vi "String to 1D Array 2.vi"(8 "Enum":T1(ring), 10 "string":string) -> (2 "Array of Strings":string[](array[string])=["sin(x)+2", "VIA(x", "y)", " VIB(z)"])   [LabVIEW 2017]
uses:
  <userlib>/_NEVSTOP/Communicable State Machine(CSM)/Communicable State Machine.lvlib
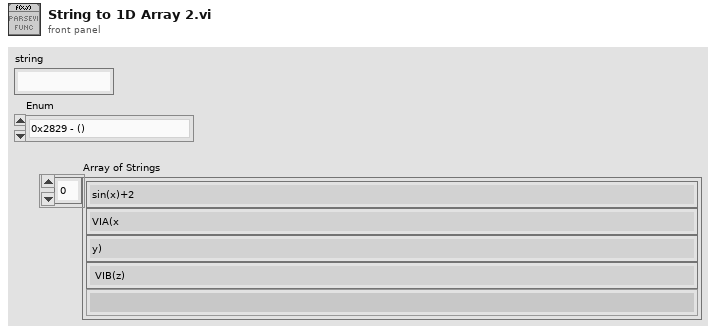
[diagram p1: front panel]
types:
  T1 = enum16{"0x2829 - ()", "0x5B5D - []", "0x7B7D - {}"}
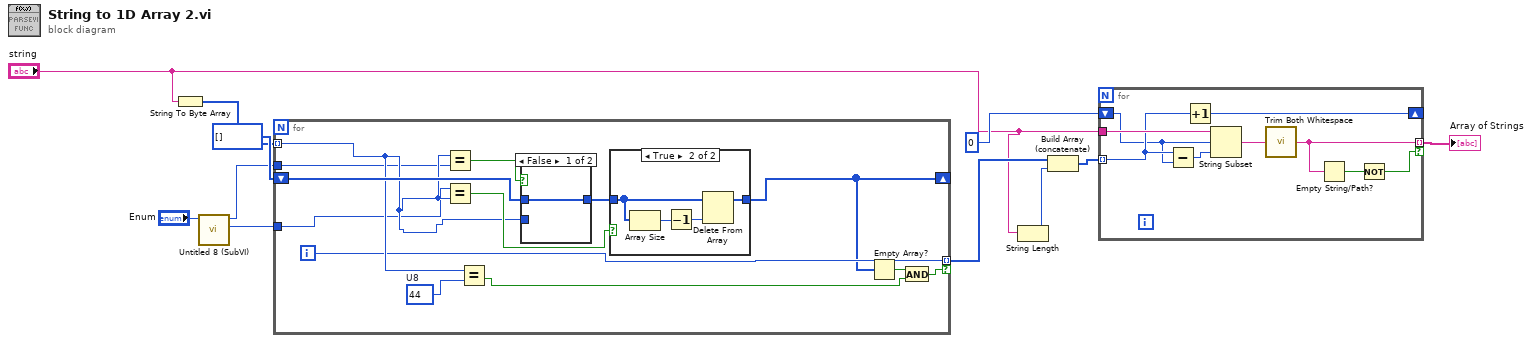
[diagram p0: block diagram]
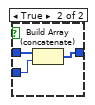
[diagram p3: hidden frame]
diagram:
  n1 = String To Byte Array(string="string") -> (unsigned byte array=w10:u8[])
  n2 = call "Untitled 8 (SubVI).vi"("Enum"="Enum") -> ("Numeric"=w1:u8, "Numeric 2"=w2:u8)  [unwired: 9 in]
  n3 = for {
    tunnel: w10 -> [w19] mode=indexing
    shift-right: [w16] -> _
    shift-left: i32[] [] -> [w21]
    tunnel: [w18] -> w9 mode=indexing if=w15
    tunnel: w2 -> [w13]
    tunnel: w1 -> [w12]
    i -> [w18]
    w20 = u8 44  # U8
    n4 = Equal?(x=w19, y=w13) -> (x = y?=w24:bool)
    n5 = Equal?(x=w12, y=w19) -> (x = y?=w22:bool)
    n6 = Equal?(x=w19, y=w20) -> (x = y?=w14:bool)
    n7 = case shown="False" w24 {
      tunnel: w21 -> [w30 w33]
      tunnel: w19 -> [_ w32]
      tunnel: [w30 w31] -> w23
      frame False {
      }
      frame True {
        n8 = Build Array (concatenate)(w33, w32) -> (w31:i32[])
      }
    }
    n9 = case shown="True" w22 {
      tunnel: w23 -> [w25 w28]
      tunnel: [w25 w26] -> w16
      frame False {
      }
      frame True {
        n10 = Array Size(array=w28) -> (size(s)=w29:i32)
        n11 = Decrement(x=w29) -> (x-1=w27:i32)
        n12 = Delete From Array(array=w28, index=w27) -> (array with subset deleted=w26:i32[])  [unwired: 1 in, 1 out]
      }
    }
    n13 = Empty Array?(array=w16) -> (empty?=w17:bool)
    n14 = And(x=w17, y=w14) -> (x .and. y?=w15:bool)
  }
  n15 = String Length(string="string") -> (length=w5:i32)
  n16 = Build Array (concatenate)(w9, w5) -> (w6:i32[])
  n17 = for {
    tunnel: "string" -> [w42]
    tunnel: w6 -> [w40] mode=indexing
    tunnel: [w36] -> w7 mode=indexing if=w34
    shift-right: [w37] -> _
    shift-left: 0 ("Numeric") -> [w38]
    n18 = Subtract(x=w40, y=w38) -> (x-y=w39:i32)
    n19 = Increment(x=w40) -> (x+1=w37:i32)
    n20 = String Subset(string=w42, offset (0)=w38, length (rest)=w39) -> (substring=w41:string)
    n21 = call <userlib>:"Trim Both Whitespace.vi"("string"=w41) -> ("trimmed string"=w36:string)  [unwired: 1 in]
    n22 = Empty String/Path?(string/path=w36) -> (empty?=w35:bool)
    n23 = Not(x=w35) -> (.not. x?=w34:bool)
  }
  "Array of Strings" <- w7
